vi "Feed Teleop.vi"(0 "Feed Wheel":bool, 1 "Reverse Feed":bool, 2 "Elevator":dbl) -> ()   [LabVIEW 2019]
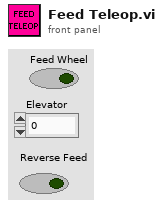
[diagram p1: front panel]
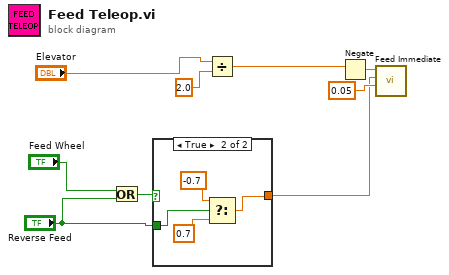
[diagram p0: block diagram]
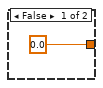
[diagram p2: hidden frame]
diagram:
  n1 = Or(x="Feed Wheel", y="Reverse Feed") -> (x .or. y?=w6:bool)
  n2 = case shown="True" w6 {
    tunnel: [0.0 w11] -> w4
    tunnel: "Reverse Feed" -> [_ w12]
    frame False {
    }
    frame True {
      n3 = Select(t=-0.7, s=w12, f=0.7) -> (s? t:f=w11:dbl)
    }
  }
  n4 = Divide(x="Elevator", y=2.0) -> (x/y=w1:dbl)
  n5 = Negate(x=w1) -> (-x=w2:dbl)
  n6 = call "Feed Immediate.vi"("Deadband Value"=0.05, "Upper Setpoint"=w4, "Lower Setpoint"=w2) -> ()  [unwired: 8 in, 1 out]
